vi "read raw default value.vi"(8 "error in":errorcluster, 11 "system tag in":refnum<class "tag descriptor.lvclass">) -> (0 "error out":errorcluster, 2 "raw default":string, 3 "system tag out":refnum<class "tag descriptor.lvclass">)   [LabVIEW 2013, in "tag bus.lvlib" / "tag descriptor.lvclass"]
doc: "Reads the default value field stored in the tag descriptor. This is returned as a raw string, not as an interpreted data type."
uses:
  tag descriptor.lvclass
  tag descriptor.lvclass/tag descriptor.ctl
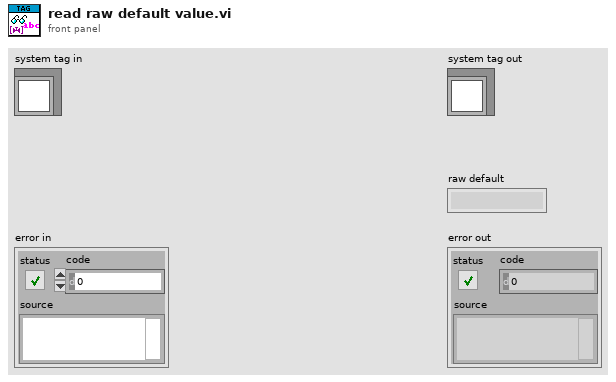
[diagram p1: front panel]
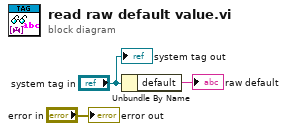
[diagram p0: block diagram]
diagram:
  n1 = Unbundle By Name("system tag in") -> ("default"=→"raw default":string)
  "system tag out" <- "system tag in"
  "error out" <- "error in"
